vi "Load Measurements from Disk.vi"(8 "error in (no error)":errorcluster, 10 "Array of paths (folders to scan or explicit files)":path[](array[path]), 11 "base path":path) -> (0 "error out":errorcluster, 2 "Available Measurements":refnum<class "Function.lvclass">[](array[class]))   [LabVIEW 2016, in "Controller Actor.lvlib" / "Controller.lvclass"]
uses:
  <userlib>/Common Components/Controller/Controller.lvclass
  <userlib>/Common Components/Function Actor/Function.lvclass
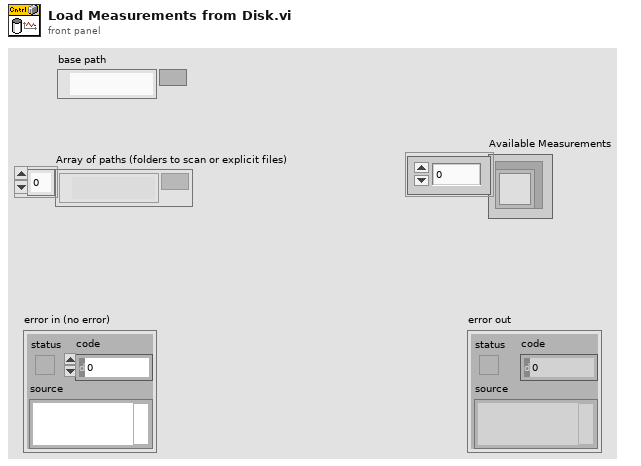
[diagram p1: front panel]
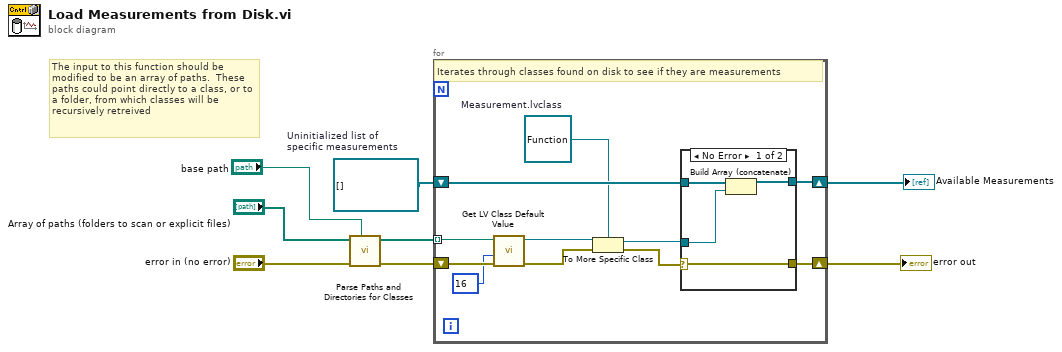
[diagram p0: block diagram]
diagram:
  w8 = refnum<class "Function.lvclass">[] []  # Uninitialized list of specific measurements
  # "The input to this function should be modified to be an array of paths.  These paths could point directly to a class, or to a folder, from which classes will be recursively retreived"
  n1 = call <userlib>:"Parse Paths and Directories for Classes.vi"("base path"="base path", "error in (no error)"="error in (no error)", "Array of paths (folders to scan or explicit files)"="Array of paths (folders to scan or explicit files)") -> ("error out"=w4:errorcluster, "All Files in Dir"=w5:path[])  [unwired: 7 in]
  n2 = for {
    shift-right: [w18] -> w7
    shift-left: w8 -> [w14]
    shift-right: [w15] -> w6
    shift-left: w4 -> [w16]
    tunnel: w5 -> [w9] mode=indexing
    w12 = refnum<class "Function.lvclass"> refnum  # Measurement.lvclass
    # "Iterates through classes found on disk to see if they are measurements"
    n3 = call <vilib>:"Get LV Class Default Value.vi"("error in (no error)"=w16, "options"=u32 16, "class path"=w9) -> ("error out"=w17:errorcluster, "object"=w13:refnum<class>)  [unwired: 7 in]
    n4 = To More Specific Class(target class=w12, reference=w13, error in=w17) -> (specific class reference=w19:refnum<class "Function.lvclass">, error out=w11:errorcluster)
    n5 = case shown="No Error" w11 {
      selector: w11 -> [w20 _]
      tunnel: w19 -> [w21 _]
      tunnel: [w23 w24] -> w18
      tunnel: w14 -> [w22 w24]
      tunnel: [w20 _] -> w15
      frame No Error {
        n6 = Build Array (concatenate)(w22, w21) -> (w23:refnum<class "Function.lvclass">[])
      }
      frame Error {
      }
    }
  }
  "error out" <- w6
  "Available Measurements" <- w7
